vi "MAIN - {TMPL} App.vi"() -> ()   [LabVIEW 2016, in "TLB` Template.lvlib" / "TLB` - {TMPL}.lvclass"]
uses:
  TLB` - {TMPL}.lvclass
  Application Components/Trigger API/{TMPL} System Trigger.ctl
  State Machine/State.ctl
  Core Components/Error Handler/TLB` Error Handler.lvclass
  Application Components/Configuration/{TMPL} Station Configuration.lvclass
  TLB` - {TMPL}.lvclass/TLB` - {TMPL}.ctl
  <vilib>/Utility/error.llb/Error Cluster From Error Code.vi
  <vilib>/ErrorRing/Error Ring.xnode
  Application Components/Trigger API/{TMPL} Trigger API.lvlib
  TLB` Template.lvlib
  Core Components/Actions/Actions.lvlib
  Core Components/Dependencies/TLB`_Dependencies.lvlib
panel:
  out "State":string
  out "Status":string
  # "TLB` Template"
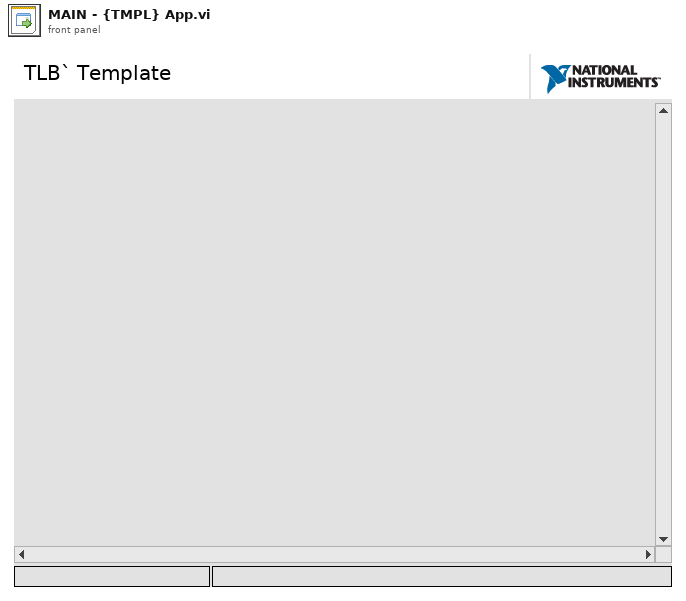
[diagram p1: front panel]
types:
  T1 = typedef "TLB` Template.lvlib/TLB` - {TMPL}.lvclass/State.ctl" = enum16{"<Startup>", "Idle", "<Shutdown>", "<Error>"}
  T2 = enum16{"Close Display", "Clear References", "Close Error Handler"}
  T3 = enum16{"Clear SR", "Set Display", "Set Shifter", "Initialize Events", "Init Q"}
  T4 = typedef "TLB` Template.lvlib/{TMPL} System Trigger.ctl" = enum16{"None", "Connect", "Start Acquisition", "Stop Acquisition", "Disconnect", "Return to Safe State Actions", "Cache User Parameters", "Close Application", "<Error>"}
  T5 = refnum<class "{TMPL} Station Configuration.lvclass">
  T6 = typedef "TLB` Template.lvlib/_UI CORE Event References.ctl" = cluster{"Exit Event":refnum<user-event>, "State Indicator":refnum<user-event>, "Status Indicator":refnum<user-event>}
  T7 = typedef "TLB` Template.lvlib/_UI APP Event References.ctl" = cluster{"Exit Event":refnum<user-event>}
  T8 = enum32{"Invalid", "Standard", "Closed", "Hidden", "Minimized", "Maximized"}
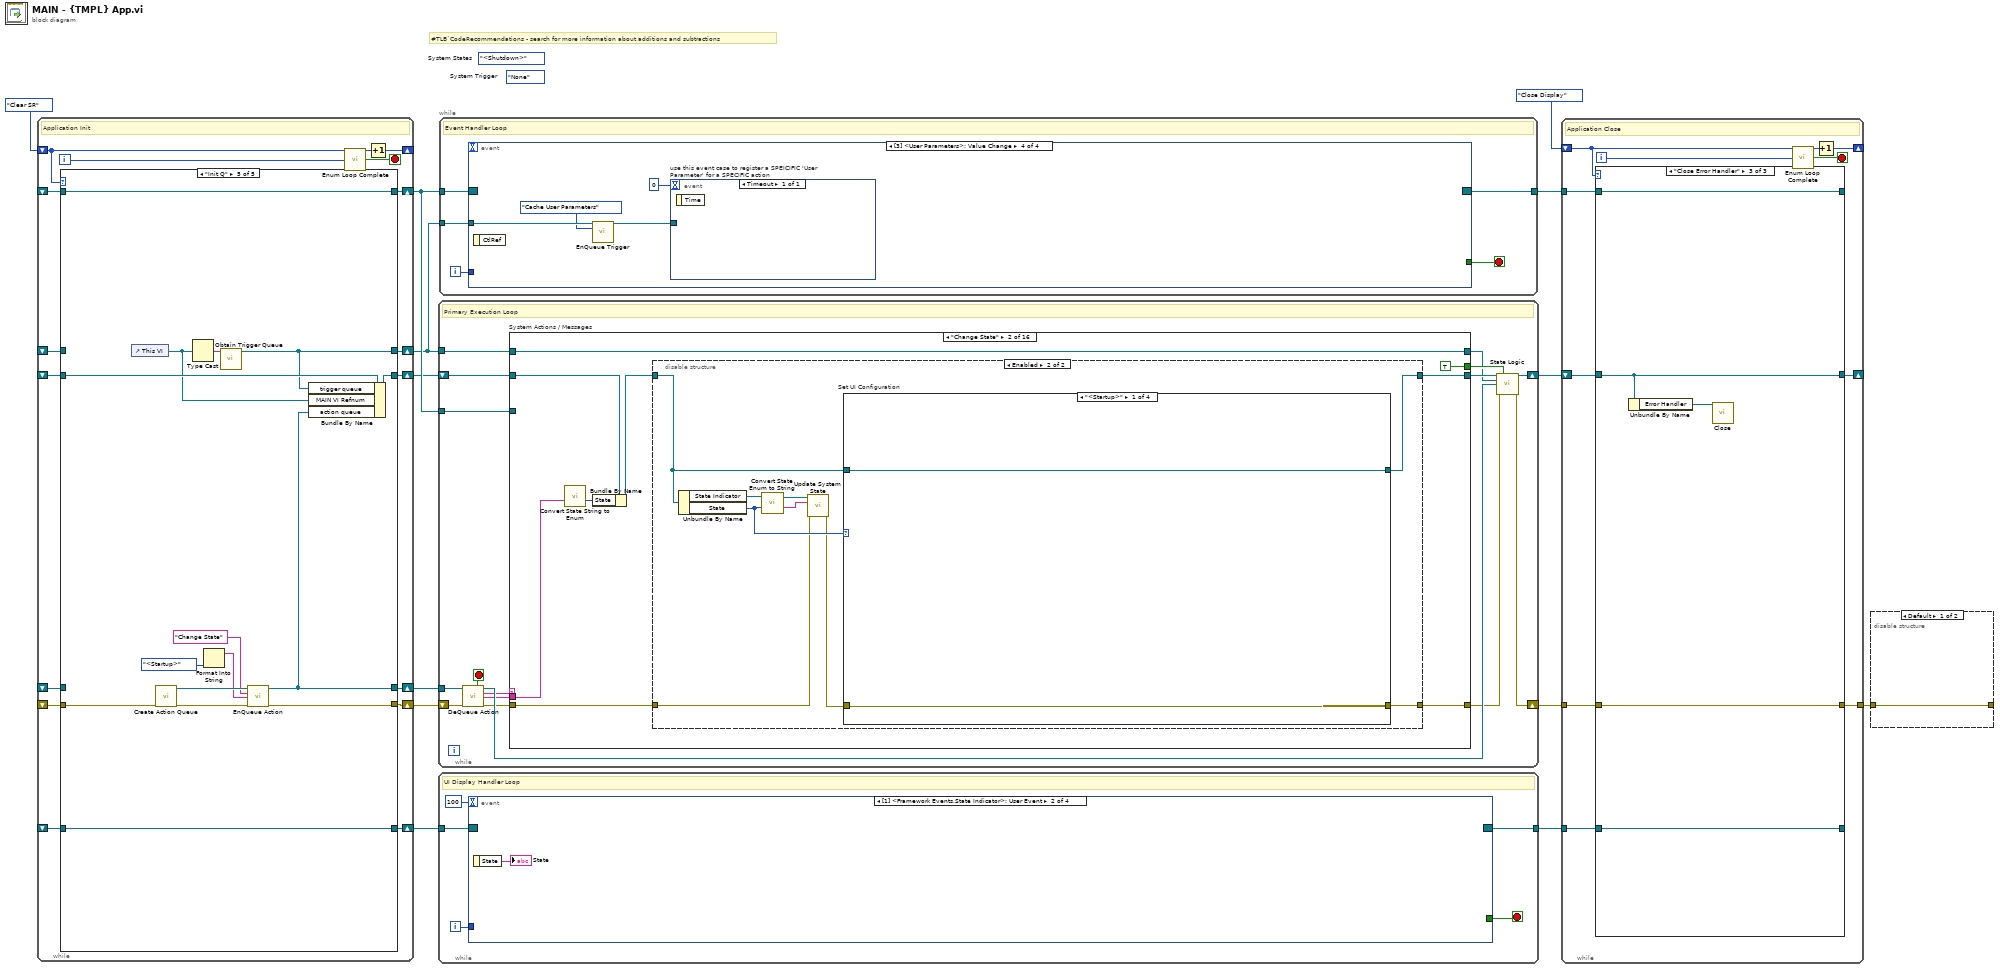
[diagram p0: block diagram]
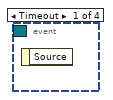
[diagram p2: hidden frame]
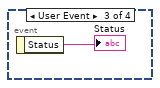
[diagram p3: hidden frame]
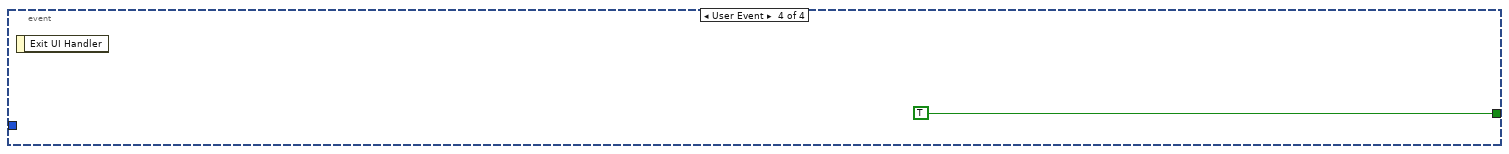
[diagram p4: hidden frame]
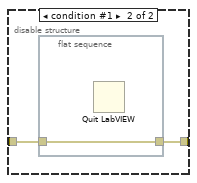
[diagram p5: hidden frame]
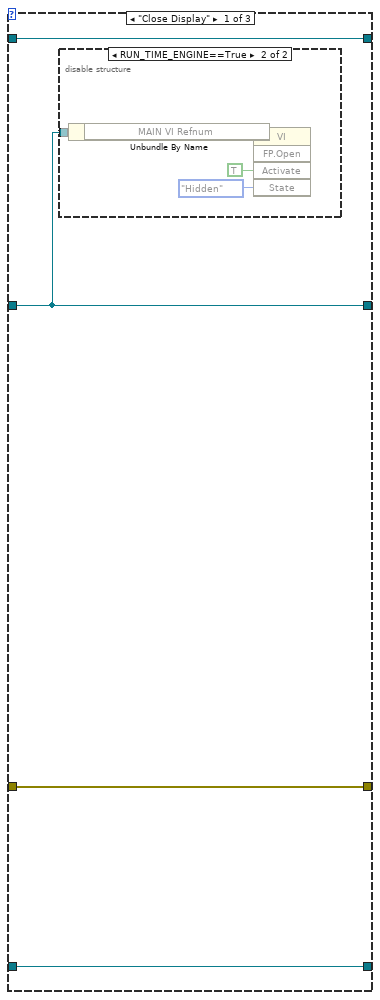
[diagram p6: hidden frame]
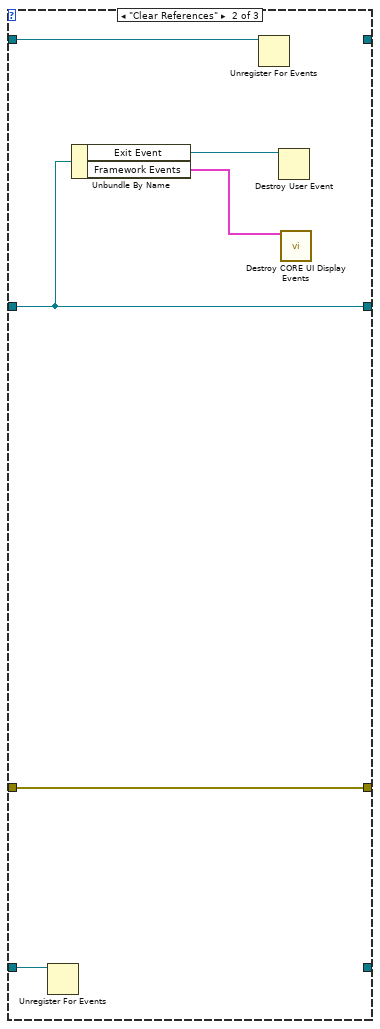
[diagram p8: hidden frame]
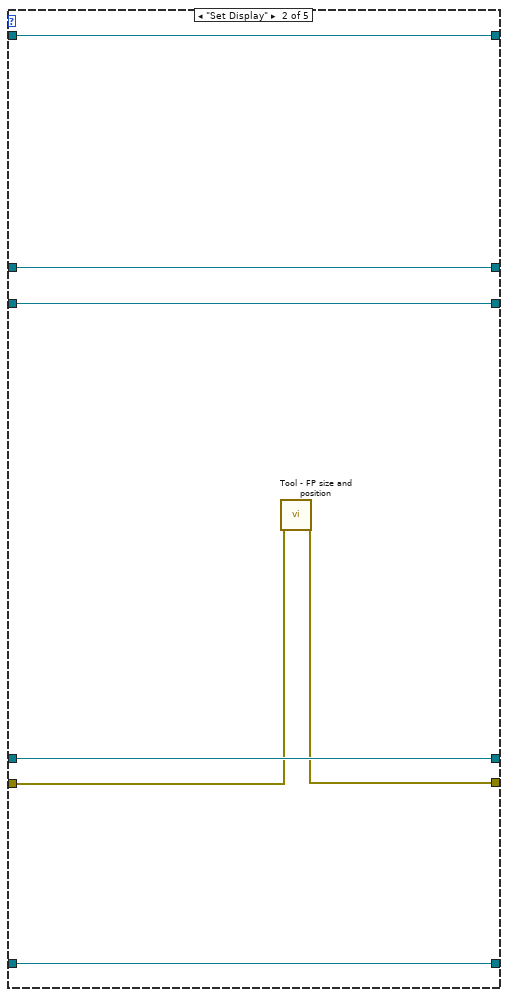
[diagram p10: hidden frame]
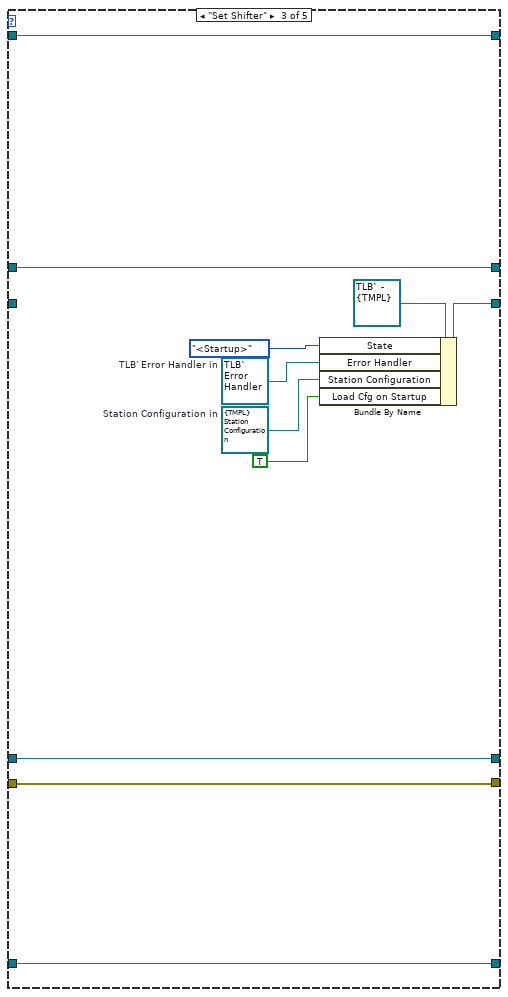
[diagram p11: hidden frame]
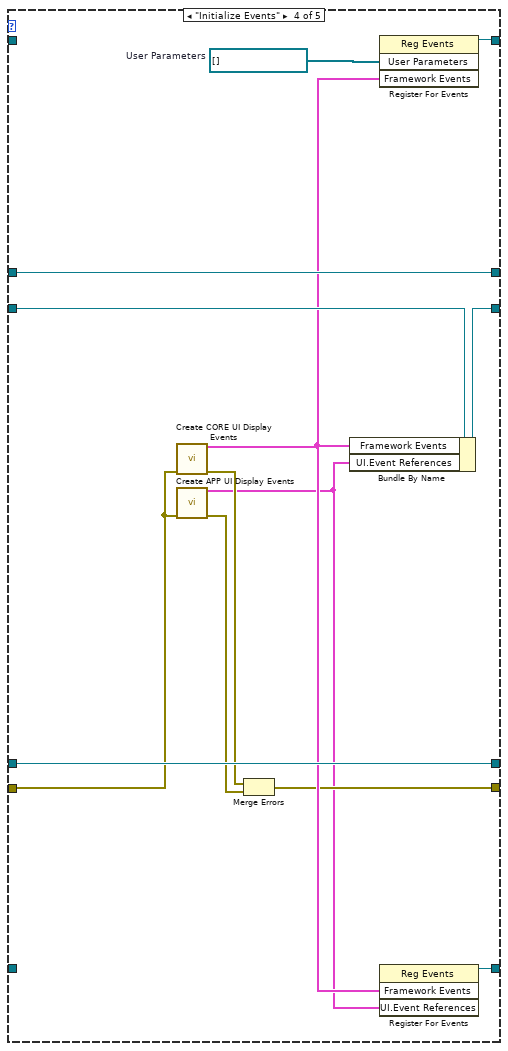
[diagram p12: hidden frame]
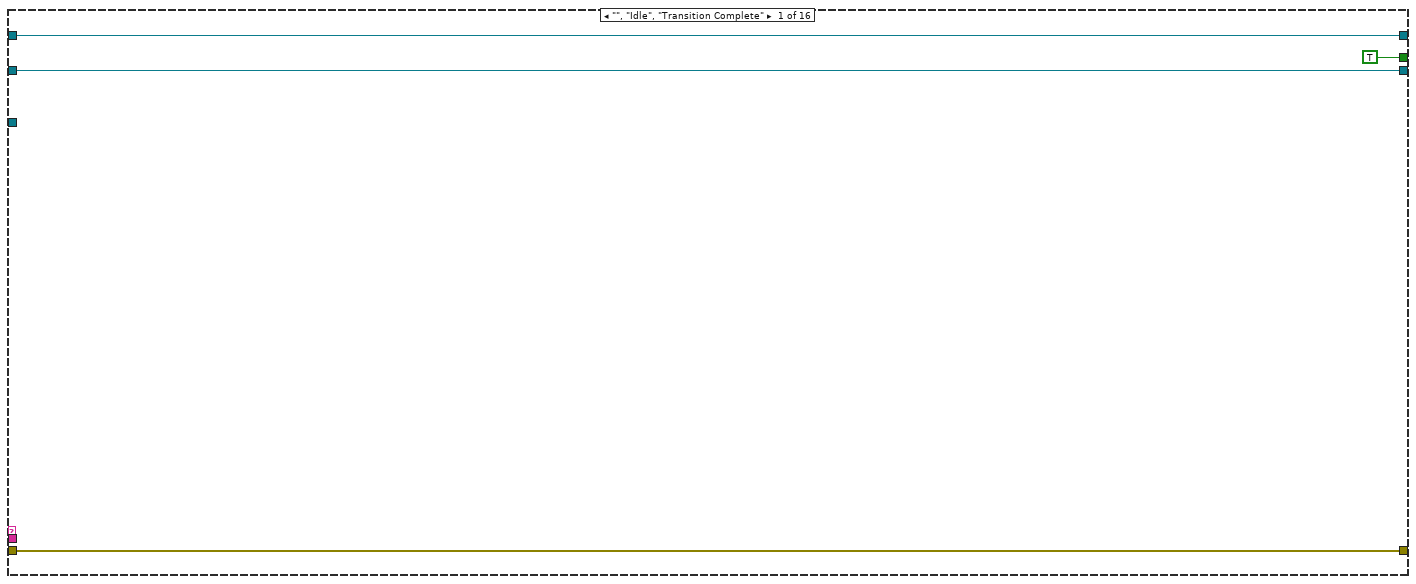
[diagram p13: hidden frame]
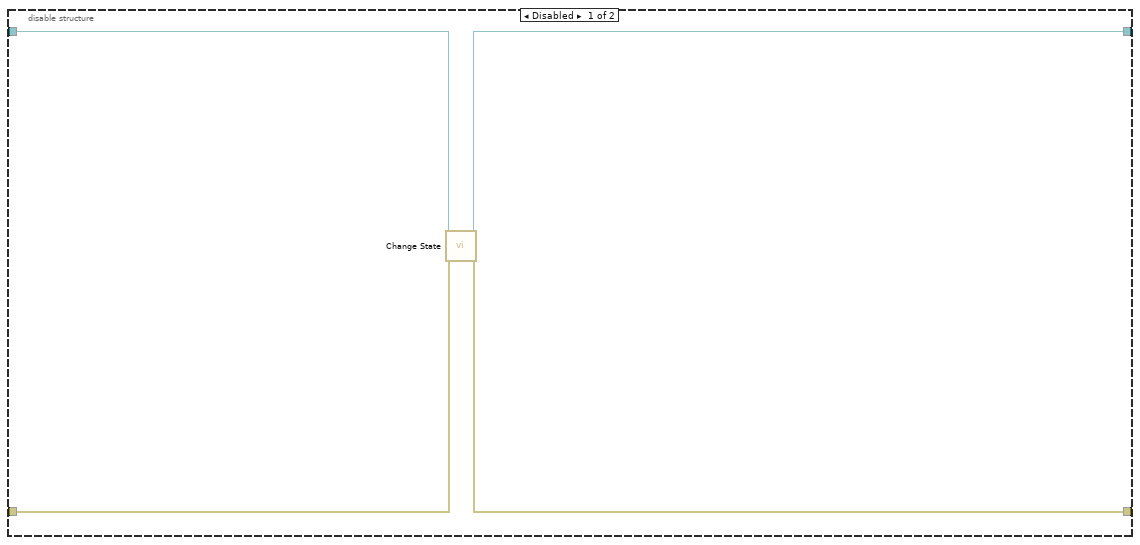
[diagram p14: hidden frame]
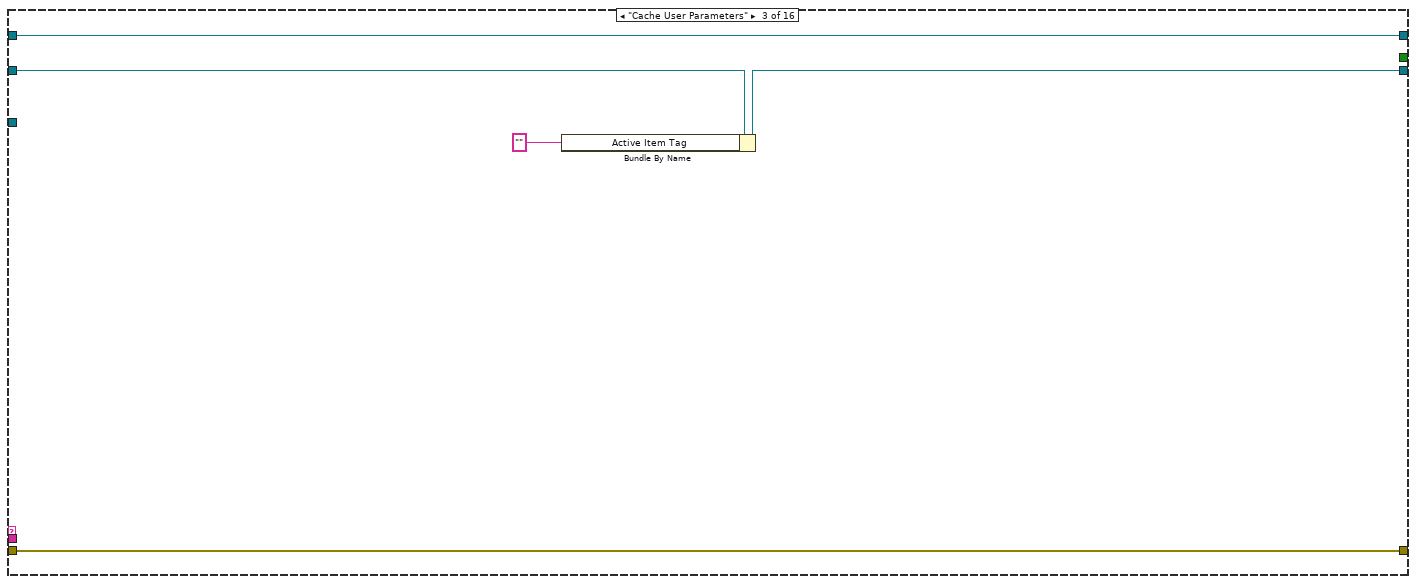
[diagram p18: hidden frame]
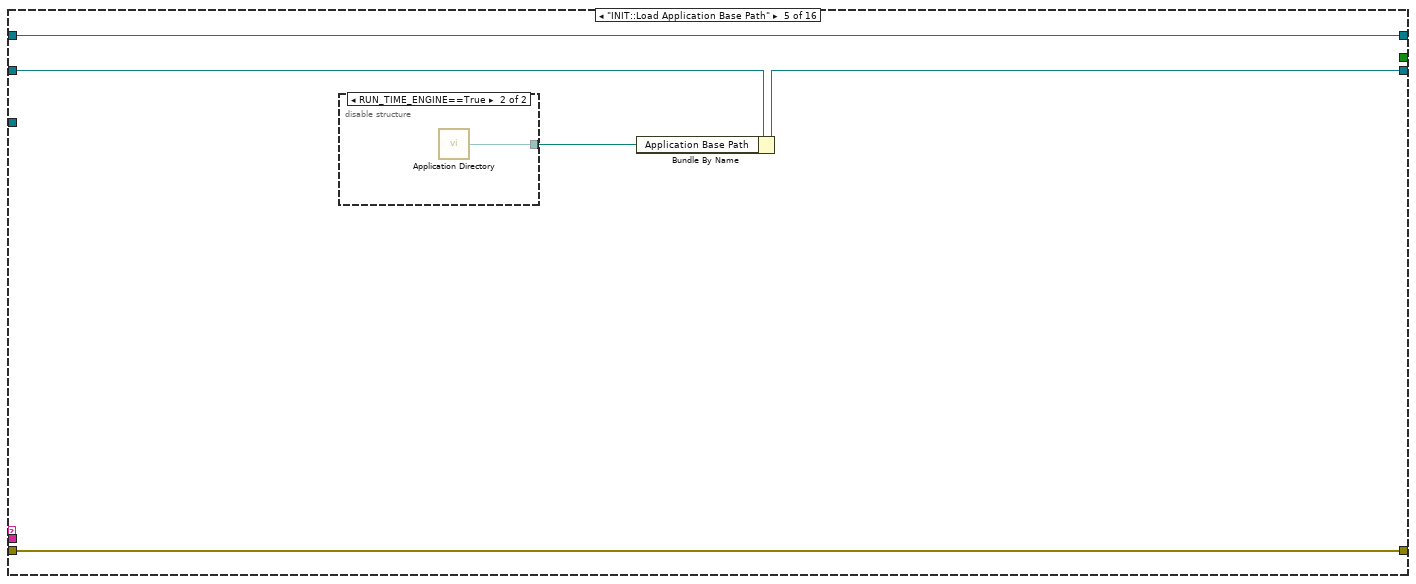
[diagram p20: hidden frame]
diagram:
  (unwired) State."<Shutdown>"  # System States
  (unwired) {TMPL}_System_Trigger."None"  # System Trigger
  # "#TLB`CodeRecommendations - search for more information about additions and subtractions"
  n1 = while {
    shift-right: [w23] -> _
    shift-left: T3."Clear SR" -> [w18]
    shift-right: [w29] -> w13
    shift-left: _ -> [w22]
    shift-right: [w26] -> w8
    shift-left: _ -> [w21]
    shift-right: [w28] -> w7
    shift-left: _ -> [w20]
    shift-right: [w27] -> w6
    shift-left: _ -> [w19]
    shift-right: [w17] -> w2
    shift-left: _ -> [w16]
    shift-right: [w15] -> w5
    shift-left: _ -> [w14]
    i -> [w24]
    stop <- w25 stop-if-true
    # "Application Init"
    n2 = case shown="\"Init Q\"" w18 {
      tunnel: [_ w34 w47 w60 w61] -> w29
      tunnel: [_ w32 w46 w50 w67] -> w26
      tunnel: [_ w36 w42 w58 w73] -> w27
      tunnel: [_ w35 w45 w57 w75] -> w28
      tunnel: w22 -> [_ w34 w47 w60 _]
      tunnel: w21 -> [_ w33 w46 w49 w69]
      tunnel: w20 -> [_ w35 w45 _ w75]
      tunnel: w19 -> [_ w36 _ w59 w74]
      tunnel: [_ w31 w44 w56 w62] -> w17
      tunnel: w16 -> [_ w31 w44 w56 _]
      tunnel: [_ w30 w40 w54 w70] -> w15
      tunnel: w14 -> [_ w30 w40 _ w70]
      frame "Clear SR" {
      }
      frame "Set Display" {
        n3 = call "Tool - FP size and position.vi"("error in (no error)"=w33) -> ("error out"=w32:errorcluster)  [unwired: 17 in, 1 out]
      }
      frame "Set Shifter" {
        w38 = T5 refnum  # Station Configuration in
        w39 = refnum<class "TLB` Error Handler.lvclass"> refnum  # TLB' Error Handler in
        n4 = Bundle By Name(cluster=refnum<class "TLB` - {TMPL}.lvclass"> refnum ("TLB` Template.lvlib:TLB' Template.lvclass"), "State"=State."<Startup>", "Error Handler"=w39, "Station Configuration"=w38, "Load Cfg on Startup"=TRUE ("Private Data.Load Cfg on Startup")) -> (w42:refnum<class "TLB` - {TMPL}.lvclass">)
      }
      frame "Initialize Events" {
        w55 = refnum<vi>[] []  # User Parameters
        n5 = call "Create CORE UI Display Events.vi"("error in"=w49) -> ("Framework Events"=w53:T6, "error out"=w52:errorcluster)  [unwired: 13 in]
        n6 = call "Create APP UI Display Events.vi"("error in"=w49) -> ("UI.Event References"=w48:T7, "error out"=w51:errorcluster)  [unwired: 13 in]
        n7 = Merge Errors(w52, w51) -> (w50:errorcluster)
        n8 = Bundle By Name(cluster=w59, "Framework Events"=w53, "UI.Event References"=w48) -> (w58:refnum<class "TLB` - {TMPL}.lvclass">)
        n9 = register-events(w55, w53) -> (reference out=w57:refnum<event-registration>)  [unwired: 2 in, 1 out]
        n10 = register-events(w53, w48) -> (reference out=w54:refnum<event-registration>)  [unwired: 2 in, 1 out]
      }
      frame "Init Q" {
        n11 = control-ref of="This VI"() -> (w72:refnum<vi>)
        n12 = call "Create Action Queue.vi"("error in"=w69) -> ("action queue out"=w66:refnum<queue>, "error out"=w68:errorcluster)  [unwired: 13 in]
        n13 = Type Cast(x=w72) -> (*(type *) &x=w63:string)  [unwired: 1 in]
        n14 = Format Into String(State."<Startup>" ("State")) -> (resulting string=w64:string)  [unwired: 3 in, 1 out]
        n15 = call "Obtain Trigger Queue.vi"("trigger queue name"=w63) -> ("trigger queue out"=w62:refnum<queue>)  [unwired: 13 in, 1 out]
        n16 = call "EnQueue Action.vi"("action queue in"=w66, "action"="Change State" ("Message Name"), "data in"=w64, "error in"=w68) -> ("action queue out"=w61:refnum<queue>, "error out"=w67:errorcluster)  [unwired: 10 in]
        n17 = Bundle By Name(cluster=w74, "trigger queue"=w62, "MAIN VI Refnum"=w72, "action queue"=w61) -> (w73:refnum<class "TLB` - {TMPL}.lvclass">)
      }
    }
    n18 = call "Enum Loop Complete.vi"("Current State Enum"=w18, "Itteration"=w24) -> ("Loop Complete?"=w25:bool)  [unwired: 12 in, 1 out]
    n19 = Increment(x=w18) -> (x+1=w23:T3)
  }
  n20 = while {
    shift-right: [w86] -> w4
    shift-left: w8 -> [w81]
    shift-right: [w88] -> w9
    shift-left: w6 -> [w90]
    tunnel: w13 -> [w82]
    tunnel: w7 -> [w89]
    tunnel: w2 -> [w85]
    stop <- w80 stop-if-true
    # "Primary Execution Loop"
    n21 = call "DeQueue Action.vi"("action queue in"=w82, "error in"=w81) -> ("exit?"=w80:bool, "action queue out"=w91:refnum<queue>, "action"=w78:string, "action value"=w76:string, "error out"=w79:errorcluster)  [unwired: 8 in, 1 out]
    n22 = case "System Actions / Messages" shown="\"Change State\"" w78 {
      selector: w78 -> [_ _ _ _ _ _ _ _ _ _ _ _ _ _ _ w225]
      tunnel: [w95 w102 w128 w132 w133 w141 w158 w174 w177 w184 w197 w202 w207 w208 w220 w224] -> w83
      tunnel: w79 -> [w95 w101 w128 w132 w133 w144 w158 w174 w177 w182 w197 w201 w207 w209 w221 _]
      tunnel: w90 -> [w92 w100 w125 w131 w136 w142 w161 w173 w176 w181 w196 w204 w206 w212 w223 w227]
      tunnel: [w92 w96 w129 w131 w135 w147 w164 w173 w176 w178 w196 w204 w206 w211 w222 w227] -> w87
      tunnel: w89 -> [_ _ _ _ _ _ w162 _ _ _ _ _ _ _ _ _]
      tunnel: [w93 w103 w127 w130 w137 w148 w163 w172 w175 w187 w195 w199 w205 w215 w216 w226] -> w77
      tunnel: w85 -> [w93 w103 w127 w130 w137 w148 w163 w172 w175 w187 w195 w199 w205 w215 w216 w226]
      tunnel: [TRUE TRUE _ _ _ _ _ _ _ _ _ _ _ _ _ _] -> w84
      tunnel: w76 -> [_ w99 _ _ _ _ _ _ _ _ _ _ _ _ _ _]
      frame "", "Idle", "Transition Complete" {
      }
      frame "Change State" {
        n23 = call "Convert State String to Enum.vi"("state in"=w99) -> ("state out"=w98:T1)  [unwired: 13 in, 1 out]
        n24 = Bundle By Name(cluster=w100, "State"=w98) -> (w97:refnum<class "TLB` - {TMPL}.lvclass">)
        n25 = disable-structure shown="Enabled" {
          disable-tunnel: [w108 w109] -> w102
          disable-tunnel: w101 -> [w107 w110]
          disable-tunnel: w97 -> [w106 w112]
          disable-tunnel: [w105 w111] -> w96
          frame Disabled {
            n26 = call "Change State.vi"("TLB' data in"=w106, "error in"=w107) -> ("TLB' data out"=w105:refnum<class "TLB` - {TMPL}.lvclass">, "error out"=w108:errorcluster)  [unwired: 12 in]
          }
          frame Enabled {
            n27 = Unbundle By Name(w112) -> ("State Indicator"=w113:refnum<user-event>, "State"=w116:T1)
            n28 = call "Convert State Enum to String.vi"("state in"=w116) -> ("state out"=w114:string)  [unwired: 13 in, 1 out]
            n29 = call "Update System State.vi"("State Indicator"=w113, "system state message"=w114, "error in"=w110) -> ("error out"=w115:errorcluster)  [unwired: 12 in]
            n30 = case "Set UI Configuration" shown="\"<Startup>\"" w116 {
              tunnel: [w117 w120 w121 w124] -> w109
              tunnel: w115 -> [w117 w120 w121 w124]
              tunnel: [w118 w119 w122 w123] -> w111
              tunnel: w112 -> [w118 w119 w122 w123]
              frame "<Startup>" {
              }
              frame "Idle" {
              }
              frame "<Error>" {
              }
              frame "<Shutdown>" {
              }
            }
          }
        }
      }
      frame "Cache User Parameters" {
        n31 = Bundle By Name(cluster=w125, "Active Item Tag"="" ("User Data.Active Item Tag")) -> (w129:refnum<class "TLB` - {TMPL}.lvclass">)
      }
      frame "/*********INITialize********/" {
      }
      frame "INIT::Load Application Base Path" {
        n32 = disable-structure shown="RUN_TIME_ENGINE==True" {
          disable-tunnel: [w138 w140] -> w134
          frame condition #0 (active) {
            n33 = Current VI's Path() -> (path=w139:path)
            n34 = Strip Path(path=w139) -> (stripped path=w138:path)  [unwired: 1 out]
          }
          frame condition #1 {
            n35 = call <vilib>:"Application Directory.vi"() -> ("Application Directory"=w140:path)
          }
        }
        n36 = Bundle By Name(cluster=w136, "Application Base Path"=w134) -> (w135:refnum<class "TLB` - {TMPL}.lvclass">)
      }
      frame "INIT::Initialize Error Handler" {
        n37 = disable-structure shown="Default" {
          disable-tunnel: [w152 w155] -> w149
          disable-tunnel: ["System Level Errors\\System Errors.txt" ("name or relative path") "System Level Errors\\System Errors.txt" ("name or relative path")] -> w150
          disable-tunnel: w142 -> [w151 w157]
          frame condition #0 (active) {
            n38 = Unbundle By Name(w151) -> ("Application Base Path"=w152:path)
          }
          frame condition #1 {
            n39 = Unbundle By Name(w157) -> ("Application Base Path"=w156:path)
            n40 = Strip Path(path=w156) -> (stripped path=w155:path)  [unwired: 1 out]
          }
        }
        n41 = Build Path(base path=w149, name or relative path=w150) -> (appended path=w145:path)
        n42 = Unbundle By Name(w142) -> ("Error Handler"=w143:refnum<class "TLB` Error Handler.lvclass">)
        n43 = call-dynamic "Open.vi"("error handler in"=w143, "error log path in"=w145, "error in"=w144) -> ("error handler out"=w146:refnum<class "TLB` Error Handler.lvclass">, "error out"=w141:errorcluster)  [unwired: 11 in]
        n44 = Bundle By Name(cluster=w142, "Error Handler"=w146) -> (w147:refnum<class "TLB` - {TMPL}.lvclass">)
      }
      frame "INIT::Register User Parameters" {
        n45 = disable-structure shown="Enabled" {
          disable-tunnel: [w165 refnum<vi>[] [] ("User Parameter Controls")] -> w160
          frame Disabled {
            n46 = stacked-sequence "Stacked Sequence Structure :: Allows for a lot of controls" {
              tunnel: [w166] -> w165
              frame #0 {
                n47 = Build Array() -> (w166:void[], w170:dbl, w169:dbl, w168:dbl, w167:dbl)
              }
            }
          }
          frame Enabled {
          }
        }
        n48 = Build Array (concatenate)(w160) -> (w159:refnum<vi>[])
        n49 = register-events(reference=w162, w159) -> ()  [unwired: 2 in, 2 out]
        n50 = Bundle By Name(cluster=w161, "User Parameter Controls"=w159) -> (w164:refnum<class "TLB` - {TMPL}.lvclass">)
      }
      frame "INIT::FP Values" {
        # "#TLB`CodeRecommendations - initialize FP values here"
      }
      frame "/*********PRImary EXEcution********/" {
      }
      frame "CFG::Load Station Configuration" {
        n51 = disable-structure shown="RUN_TIME_ENGINE==True" {
          disable-tunnel: [w189 w192] -> w186
          disable-tunnel: ["System Configuration\\Station Configuration.ini" ("name or relative path") "System Configuration\\Station Configuration.ini" ("name or relative path")] -> w185
          disable-tunnel: w181 -> [w188 w193]
          frame condition #0 (active) {
            n52 = Unbundle By Name(w188) -> ("Application Base Path"=w189:path)
          }
          frame condition #1 {
            n53 = Unbundle By Name(w193) -> ("Application Base Path"=w194:path)
            n54 = Strip Path(path=w194) -> (stripped path=w192:path)  [unwired: 1 out]
          }
        }
        n55 = Build Path(base path=w186, name or relative path=w185) -> (appended path=w183:path)
        n56 = Unbundle By Name(w181) -> ("Station Configuration"=w180:T5)
        n57 = call-dynamic "Load Configuration.vi"("INI Station Configuration in"=w180, "INI file path in"=w183, "error in"=w182) -> ("INI Station Configuration out"=w179:T5, "error out"=w184:errorcluster)  [unwired: 11 in]
        n58 = Bundle By Name(cluster=w181, "Station Configuration"=w179) -> (w178:refnum<class "TLB` - {TMPL}.lvclass">)
      }
      frame "/*********SHUTDOWN********/" {
      }
      frame "Exit" {
        w200 = refnum<class> refnum  # event data
        # "Don't wire 'Error In'\nMust Execute Regardless"
        n59 = Unbundle By Name(w204) -> ("Exit Event"=w198:refnum<user-event>)
        n60 = Generate User Event(user event=w198, event data cluster=w200) -> (error out=w203:errorcluster)  [unwired: 2 in, 1 out]
        n61 = Merge Errors(w201, w203) -> (w202:errorcluster)
      }
      frame "/*********ERRor Handler********/" {
      }
      frame "ERR::Log" {
        n62 = Unbundle By Name(w212) -> ("Error Handler"=w214:refnum<class "TLB` Error Handler.lvclass">)
        n63 = call-dynamic "Log.vi"("error handler in"=w214) -> ("error handler out"=w213:refnum<class "TLB` Error Handler.lvclass">, "error out"=w210:errorcluster)  [unwired: 13 in]
        n64 = Bundle By Name(cluster=w212, "Error Handler"=w213) -> (w211:refnum<class "TLB` - {TMPL}.lvclass">)
        n65 = Merge Errors(w209, w210) -> (w208:errorcluster)
      }
      frame "ERR::Dialog" {
        n66 = Unbundle By Name(w223) -> ("Error Handler"=w219:refnum<class "TLB` Error Handler.lvclass">)
        n67 = call-dynamic "Dialog.vi"("error handler in"=w219, "trigger queue in"=w216) -> ("error handler out"=w218:refnum<class "TLB` Error Handler.lvclass">, "error out"=w217:errorcluster)  [unwired: 12 in]
        n68 = Merge Errors(w221, w217) -> (w220:errorcluster)
        n69 = Bundle By Name(cluster=w223, "Error Handler"=w218) -> (w222:refnum<class "TLB` - {TMPL}.lvclass">)
      }
      frame Default {
        n70 = xnode "Error Ring"("parameter 0"=w225) -> ("error out"=w224:errorcluster)
      }
    }
    n71 = call "State Logic.vi"("TLB' data in"=w87, "process state logic enable"=w84, "trigger queue in"=w77, "action queue in"=w91, "error in"=w83) -> ("TLB' data out"=w88:refnum<class "TLB` - {TMPL}.lvclass">, "error out"=w86:errorcluster)  [unwired: 9 in]
  }
  n72 = while {
    tunnel: w5 -> [w239]
    tunnel: [w235] -> w3
    i -> [w238]
    stop <- w237 stop-if-true
    # "UI Display Handler Loop"
    n73 = event shown="[1] <Framework Events.State Indicator>: User Event" {
      selector: w239 -> [_ _ _ _]
      dyn-events: [_ _ _ _] -> w235
      timeout: 100 -> [_ _ _ _]
      tunnel: w238 -> [_ _ _ _]
      tunnel: [_ _ _ TRUE] -> w237
      event Timeout {
        n74 = event-data() -> ()  [unwired: 2 out]
      }
      event User Event {
        n75 = event-data() -> ("State"=→"State":string)  [unwired: 1 out]
      }
      event User Event {
        n76 = event-data() -> ("Status"=→"Status":string)  [unwired: 1 out]
      }
      event User Event {
        n77 = event-data() -> ()  [unwired: 2 out]
      }
    }
  }
  n78 = while {
    tunnel: w7 -> [w246]
    tunnel: [w245] -> w10
    tunnel: w2 -> [w243]
    i -> [w244]
    stop <- w247 stop-if-true
    # "Event Handler Loop"
    n79 = event shown="[3] <User Parameters>: Value Change" {
      selector: w246 -> [_ _ _ _]
      dyn-events: [_ _ _ _] -> w245
      timeout: _ -> [_ _ _ _]
      tunnel: [_ _ TRUE ("NewVal") _] -> w247
      tunnel: w244 -> [_ _ _ _]
      tunnel: w243 -> [w248 _ w261 w265]
      event Panel Close? {
        w250 = TRUE  # Discard?
        n80 = event-data() -> ()  [unwired: 2 out]
        n81 = call "EnQueue Trigger.vi"("trigger queue in"=w248, "system trigger"={TMPL}_System_Trigger."Close Application" ("System Trigger")) -> ()  [unwired: 12 in, 2 out]
        n82 = event-data("Discard?"=w250) -> ()  [unwired: 1 in, 1 out]
      }
      event Mouse Down {
        n83 = event-data() -> ("Button"=w255:u16, "Mods"=w256:cluster{"Double Click":bool, "Menu Key":bool})  [unwired: 1 out]
        n84 = Unbundle By Name(w256) -> ("Double Click"=w252:bool)
        n85 = Equal?(x=u16 2, y=w255) -> (x = y?=w253:bool)
        n86 = Compound Arithmetic op=AND(w253, w252) -> (w251:bool)
        n87 = case "Toggle Menu Visibility :: double RIGHT click on logo" shown="True" w251 {
          frame False {
          }
          frame True {
            n88 = property class="VI"() -> (reference out=w259:refnum<vi>, "TB.Visible"=w257:bool)  [unwired: 2 in, 1 out]
            n89 = Not(x=w257) -> (.not. x?=w258:bool)
            n90 = property class="VI"(reference=w259, "TB.Visible"=w258) -> ()  [unwired: 1 in, 2 out]
          }
        }
      }
      event User Event {
        n91 = event-data() -> ()  [unwired: 2 out]
        n92 = call "EnQueue Trigger.vi"("trigger queue in"=w261, "system trigger"={TMPL}_System_Trigger."Close Application" ("System Trigger")) -> ()  [unwired: 12 in, 2 out]
      }
      event Value Change {
        n93 = event-data() -> ()  [unwired: 2 out]
        n94 = call "EnQueue Trigger.vi"("trigger queue in"=w265, "system trigger"={TMPL}_System_Trigger."Cache User Parameters" ("System Trigger")) -> ("trigger queue out"=w264:refnum<queue>)  [unwired: 12 in, 1 out]
        n95 = event "use this event case to register a SPEICIFIC 'User Parameter' for a SPECIFIC action" shown="[0] Timeout" {
          selector: _ -> [_]
          dyn-events: _ -> [_]
          timeout: 0 -> [_]
          tunnel: w264 -> [_]
          event Timeout {
            n96 = event-data() -> ()  [unwired: 1 in, 1 out]
          }
        }
      }
    }
  }
  n97 = while {
    shift-right: [w274] -> _
    shift-left: T2."Close Display" -> [w273]
    tunnel: w10 -> [w271]
    tunnel: w4 -> [w272]
    tunnel: [w269] -> w12
    shift-right: [w268] -> _
    shift-left: w9 -> [w270]
    tunnel: w3 -> [w267]
    i -> [w275]
    stop <- w276 stop-if-true
    # "Application Close"
    n98 = case shown="\"Close Error Handler\"" w273 {
      tunnel: [w279 w290 w295] -> w269
      tunnel: [w278 w289 w292] -> w268
      tunnel: [w280 _ w294] -> _
      tunnel: w272 -> [w279 w290 w295]
      tunnel: w271 -> [w280 w287 w294]
      tunnel: w270 -> [w278 w289 w292]
      tunnel: w267 -> [w277 w285 w293]
      tunnel: [w277 _ w293] -> _
      frame "Close Display" {
        n99 = disable-structure shown="RUN_TIME_ENGINE==True" {
          disable-tunnel: w278 -> [_ w282]
          frame condition #0 (active) {
          }
          frame condition #1 {
            n100 = Unbundle By Name(w282) -> ("MAIN VI Refnum"=w281:refnum<vi>)
            n101 = invoke class="VI" method="FP.Open"(reference=w281, "Activate"=TRUE ("Activate?"), "State"=T8."Hidden") -> ()  [unwired: 2 in, 5 out]
          }
        }
      }
      frame "Clear References" {
        n102 = Unregister For Events(event registration refnum=w285) -> ()  [unwired: 1 in, 1 out]
        n103 = Unbundle By Name(w289) -> ("Exit Event"=w288:refnum<user-event>, "Framework Events"=w286:T6)
        n104 = Unregister For Events(event registration refnum=w287) -> ()  [unwired: 1 in, 1 out]
        n105 = Destroy User Event(user event=w288) -> ()  [unwired: 1 in, 1 out]
        n106 = call "Destroy CORE UI Display Events.vi"("UI display events in"=w286) -> ()  [unwired: 14 in, 1 out]
      }
      frame "Close Error Handler" {
        n107 = Unbundle By Name(w292) -> ("Error Handler"=w291:refnum<class "TLB` Error Handler.lvclass">)
        n108 = call-dynamic "Close.vi"("error handler in"=w291) -> ()  [unwired: 14 in, 1 out]
      }
    }
    n109 = call "Enum Loop Complete.vi"("Current State Enum"=w273, "Itteration"=w275) -> ("Loop Complete?"=w276:bool)  [unwired: 12 in, 1 out]
    n110 = Increment(x=w273) -> (x+1=w274:T2)
  }
  n111 = disable-structure shown="Default" {
    disable-tunnel: [w296 w297] -> _
    disable-tunnel: w12 -> [w296 w298]
    frame condition #0 (active) {
    }
    frame condition #1 {
      n112 = flat-sequence {
        tunnel: [w299] -> w297
        tunnel: w298 -> [w299]
        frame #0 {
          n113 = Quit LabVIEW() -> ()  [unwired: 1 in]
        }
      }
    }
  }
